vi "AddDataListener.vi"(8 "error in (no error)":errorcluster, 9 "Listener In":refnum<class "Message Enqueuer.lvclass">, 10 "Label":string, 11 "Analyser in":refnum<class "Analyser.lvclass">) -> (0 "error out":errorcluster, 3 "Analyser out":refnum<class "Analyser.lvclass">)   [LabVIEW 2020, in "Analyser.lvlib" / "Analyser.lvclass"]
uses:
  Analyser.lvclass
  <vilib>/ActorFramework/Message Enqueuer/Message Enqueuer.lvclass
  Analyser.lvclass/Analyser.ctl
panel:
  out "key already included?":bool
  out "value unchanged?":bool
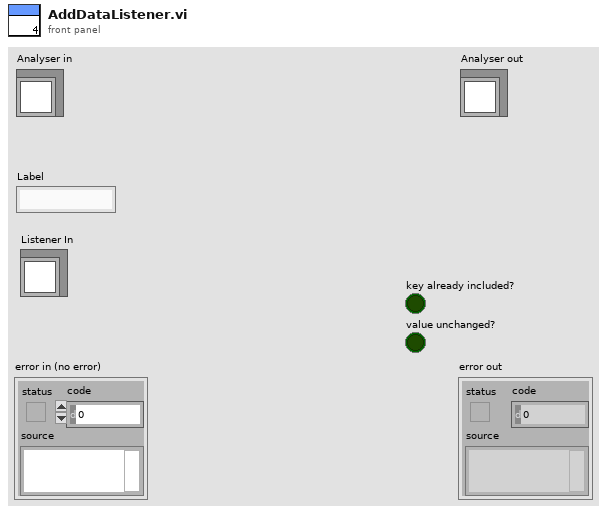
[diagram p1: front panel]
types:
  T1 = map{string, refnum<class "Message Enqueuer.lvclass">}
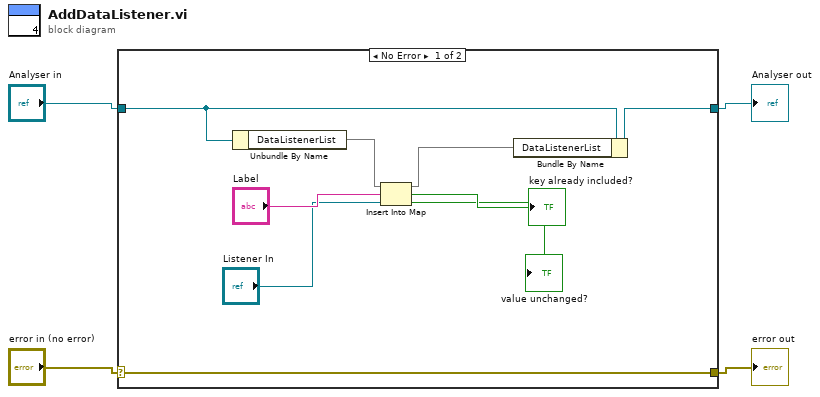
[diagram p0: block diagram]
diagram:
  n1 = case shown="No Error" "error in (no error)" {
    selector: "error in (no error)" -> [w13 w15]
    tunnel: [w13 w15] -> w2
    tunnel: [w12 w14] -> w1
    tunnel: "Analyser in" -> [w11 w14]
    frame No Error {
      n2 = Unbundle By Name(w11) -> ("DataListenerList"=w10:T1)
      n3 = Insert Into Map(map in=w10, key="Label", value="Listener In") -> (map out=w7:T1, key already included?=→"key already included?":bool, value unchanged?=→"value unchanged?":bool)
      n4 = Bundle By Name(cluster=w11, "DataListenerList"=w7) -> (w12:refnum<class "Analyser.lvclass">)
    }
    frame Error {
    }
  }
  "error out" <- w2
  "Analyser out" <- w1
